vi "Log UUT Operational Time.vi"(8 "error in (no error)":errorcluster, 11 "Report in":refnum<class "Report.lvclass">) -> (0 "error out":errorcluster, 3 "Report out":refnum<class "Report.lvclass">)   [LabVIEW 2019]
uses:
  Report.lvclass
  Custom Controls/Report Action.ctl
  PPL/Chronometer.lvlibp/Chronometer.lvclass
  C:/Users/rdexter/Documents/Development/Drivers/PPL/Instruments.lvlibp/Instruments.lvclass
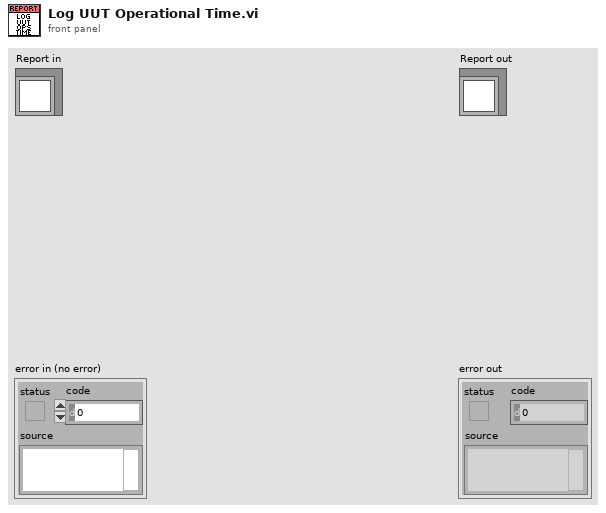
[diagram p1: front panel]
types:
  T1 = typedef "Report.lvlib/Report.lvclass/Report Action.ctl" = enum16{"Create", "Append", "Destroy"}
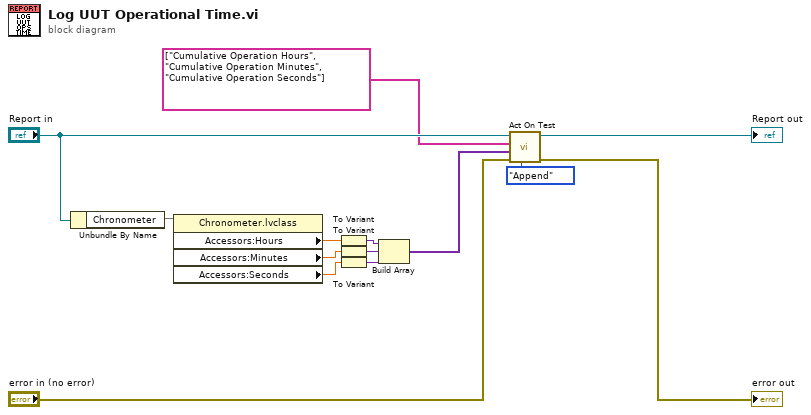
[diagram p0: block diagram]
diagram:
  n1 = Unbundle By Name("Report in") -> ("Chronometer"=w14)
  n2 = property class="Chronometer.lvclass"(reference=w14) -> ("Accessors:Hours"=w3:dbl, "Accessors:Minutes"=w2:dbl, "Accessors:Seconds"=w1:dbl)  [unwired: 1 in, 2 out]
  n3 = To Variant(anything=w3) -> (Variant=w7:variant)
  n4 = To Variant(anything=w2) -> (Variant=w5:variant)
  n5 = To Variant(anything=w1) -> (Variant=w4:variant)
  n6 = Build Array(w7, w5, w4) -> (w6:variant[])
  n7 = call-dynamic "Act On Test.vi"("Report Action"=Report_Action."Append", "error in (no error)"="error in (no error)", "Values"=w6, "Parameters"=string[] ["Cumulative Operation Hours", "Cumulative Operation Minutes", "Cumulative Operation Seconds"], "Report in"="Report in") -> ("error out"=→"error out":errorcluster, "Report out"=→"Report out":refnum<class "Report.lvclass">)  [unwired: 5 in]
